vi "ncAFM Amplitude Calibration.vi"() -> ()   [LabVIEW 2021]
doc: "This example calculates the amplitude calibration in non-contact AFM mode.\n\nThis routine is explained in detail in the \"Automated Amplitude Calibration In non-contact AFM\" application note which can be found in www.specs-zurich.com.\n\n\n- Nanonis Programming Interface -"
uses:
  Nanonis Prog Interface.lvlib
  <vilib>/Analysis/NI_AALPro.lvlib
  <vilib>/Analysis/NI_AALBase.lvlib
  <vilib>/Utility/config.llb/NI_LVConfig.lvlib
  <vilib>/Utility/config.llb/Write Key (Double).vi
  Instance           1 35Saved   ncAFM Amplitude Calibration .vi
panel:
  out "Initial P-gain":sgl
  in  "Finish":bool
  in  "apply calib":bool
  out "Initial Z-Controller\nsetpoint [Hz]":sgl format="%.2p"
  out "Initial amplitude A [m]":sgl format="%.2p"
  in  "Tip lift [m]":sgl format="%.2p"
  out "Standard deviation":dbl format="%.2p"
  out "Mean calibration  [m/V]":dbl format="%.2p"
  out "Calibration":cluster{i32[], dbl[]}(graph)
  in  "No. sweeps":i32
  in  "DA [m]":dbl format="%.2p"
  out "Initial calibration [m/V]":sgl format="%.2p"
  in  "Choose PLL":enum16{"PLL1", "PLL2"}(ring)=enum."PLL2"
  in  "No. Points":i32=10
  out "Z versus Amplitude":cluster{dbl[], "Best Linear Fit":dbl[]}[](graph)
  out "Gamma":dbl format="%.2p"
  in  "Machine name (localhost)":string="localhost"
  # "Amplitude calibration in nc-AFM\n\nUser input parameters:  The user should set up the PLL before the calibration procedure.  The amplitude setpoint in Oscillator Controller (A) and the setpoint of the Z-controller (Df) have to be setup to  values the user used to work with (approach or scan). Then the desired PLL has to be selected (useful for Dual-OC4 users).  The maximum amplitude range for sweeping the amplitude has to be also specified by the users (A±DA). \"no. Points\" defines the sweeping points for the amplitude in the range 2DA, and \"no of sweeps\" is the repetition number of the sweeping process.  When the calibration is calculated and applied the tip has to be lifted up; the user has to set in the begining the \"Tip lift\".\nMake sure the tip is engaged and then run the vi.\n\nRead initial settings: The program returns the actual amplitude (A) , the current calibration,  the current Df and calculates the changing factor gamma.\n\nAveraged calibration:  After the calibration procedure is repeated \" no. sweeps\" times , the mean calibration [m/V]  and the standard deviation are returned.\nWhen the mean calibration is calculated the user has to press either the \"Apply calibration\" button or the \"Finish\" button.\n\nThis routine is explained in detail in the \"Automated Amplitude Calibration In non-contact AFM\" application note which can be found in the Applications section of www.specs-zurich.com."
  # "User input parameters"
  # "Read initial settings"
  # "Averaged calibration"
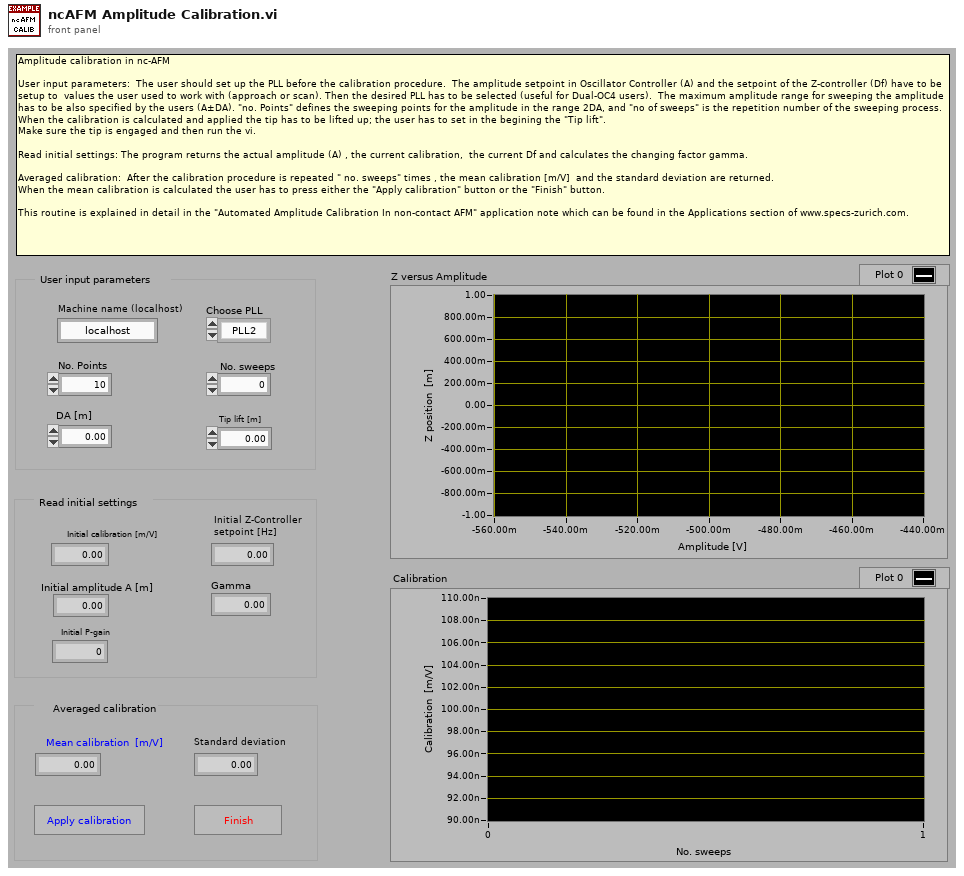
[diagram p1: front panel]
types:
  T1 = typedef "NI_LVConfig.lvlib/Config Data RefNum.ctl" = refnum<k1>
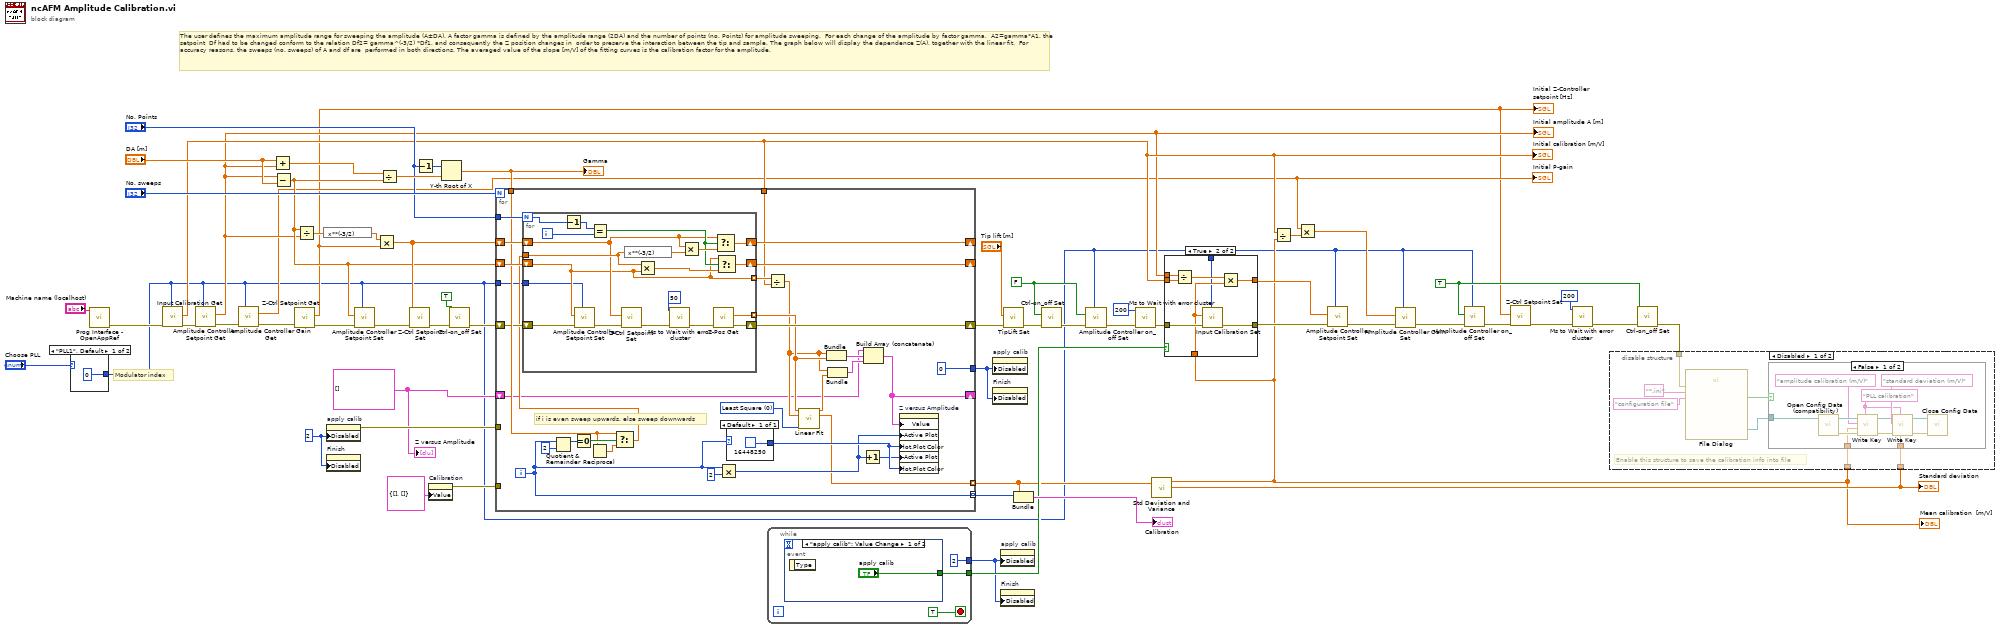
[diagram p0: block diagram]
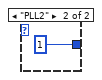
[diagram p2: hidden frame]
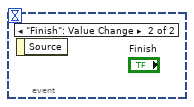
[diagram p5: hidden frame]
diagram:
  w40 = u8 2 ("Disabled")
  w27 = cluster{dbl[], "Best Linear Fit":dbl[]}[] [] ("appended array")
  w18 = TRUE
  w19 = FALSE
  # "Modulator index"
  # "The user defines the maximum amplitude range for sweeping the amplitude (A±DA). A factor gamma is defined by the amplitude range (2DA) and the number of points (no. Points) for amplitude sweeping.  For each change of the amplitude by factor gamma,  A2=gamma*A1, the setpoint  Df had to be changed conform to the relation Df2= gamma^(-3/2) *Df1, and consequently the Z position changes in  order to preserve the interaction between the tip and sample. The graph below will display the dependence Z(A), together with the linear fit.  For accuracy reasons, the sweeps (no. sweeps) of A and df are  performed in both directions. The averaged value of the slope [m/V] of the fitting curves is the calibration factor for the amplitude."
  n1 = case shown="\"PLL1\", Default" "Choose PLL" {
    tunnel: [0 ("Modulator index") 1 ("Modulator index")] -> w3
    frame "PLL1", Default {
    }
    frame "PLL2" {
    }
  }
  n2 = call <userlib>:"Prog Interface - OpenAppRef.vi"("Machine name (local machine IP)"="Machine name (localhost)") -> ("Error out"=w16:errorcluster)  [unwired: 5 in, 1 out]
  n3 = call <userlib>:"Input Calibration Get.vi"("Modulator index"=w3, "Error in (no error)"=w16) -> ("Error out"=w4:errorcluster, "Calibration (m/V)"=w15:sgl)  [unwired: 7 in, 1 out]
  "Initial calibration [m/V]" <- w15
  n4 = call <userlib>:"Amplitude Controller Setpoint Get.vi"("Modulator index"=w3, "Error in (no error)"=w4) -> ("Error out"=w5:errorcluster, "Amplitude (m)"=w14:sgl)  [unwired: 7 in, 1 out]
  "Initial amplitude A [m]" <- w14
  n5 = call <userlib>:"Amplitude Controller Gain Get.vi"("Modulator index"=w3, "Error in (no error)"=w5) -> ("P-gain (V/m)"=w13:sgl, "Error out"=w17:errorcluster)  [unwired: 9 in, 3 out]
  "Initial P-gain" <- w13
  n6 = Add(x="DA [m]", y=w14) -> (x+y=w48:dbl)
  n7 = Subtract(x=w14, y="DA [m]") -> (x-y=w34:dbl)
  n8 = call <userlib>:"Z-Ctrl Setpoint Get.vi"("error in (no error)"=w17) -> ("error out"=w44:errorcluster, "Z Controller setpoint"=w10:sgl)  [unwired: 7 in, 1 out]
  "Initial Z-Controller\nsetpoint [Hz]" <- w10
  n9 = Divide(x=w34, y=w14) -> (x/y=w47:dbl)
  n10 = expression code="x**(-3/2)"(w47) -> (w46:dbl)
  n11 = property on="apply calib" class="Bool"("Disabled"=w40) -> (error out=w39:errorcluster)  [unwired: 2 in, 1 out]
  n12 = property on="Finish" class="Bool"("Disabled"=w40) -> ()  [unwired: 2 in, 2 out]
  n13 = call <userlib>:"Amplitude Controller Setpoint Set.vi"("Modulator index"=w3, "Error in (no error)"=w44, "Amplitude (m)"=w34) -> ("Error out"=w45:errorcluster)  [unwired: 7 in, 1 out]
  n14 = Multiply(x=w46, y=w10) -> (x*y=w43:dbl)
  n15 = Divide(x=w48, y=w34) -> (x/y=w57:dbl)
  n16 = call <userlib>:"Z-Ctrl Setpoint Set.vi"("error in (no error)"=w45, "Z Controller setpoint"=w43) -> ("error out"=w60:errorcluster)  [unwired: 8 in, 1 out]
  n17 = Decrement(x="No. Points") -> (x-1=w56:i32)
  n18 = property on="Calibration" class="XYGraph (strict)"("Value"=cluster{i32[], dbl[]} {[], []} ("Calibration")) -> (error out=w25:errorcluster)  [unwired: 2 in, 1 out]
  n19 = Y-th Root of X(1:w57, 2:w56) -> (0:w55:dbl)
  "Gamma" <- w55
  n20 = call <userlib>:"Ctrl-on_off Set.vi"("error in (no error)"=w60, "Z Controller ON/OFF"=TRUE) -> ("error out"=w31:errorcluster)  [unwired: 8 in, 1 out]
  n21 = for {
    N: "No. sweeps" -> [_]
    tunnel: "No. Points" -> [w89]
    tunnel: w55 -> [w84]
    shift-right: [w81] -> w29
    shift-left: w31 -> [w80]
    shift-right: [w78] -> _
    shift-left: w43 -> [w90]
    shift-right: [w77] -> _
    shift-left: w34 -> [w88]
    tunnel: w15 -> [w75]
    shift-right: [w67] -> _
    shift-left: w27 -> [w72]
    tunnel: w39 -> [_]
    tunnel: [u8 0 ("Disabled")] -> w38
    tunnel: [w65] -> w36 mode=indexing
    tunnel: [w64] -> w35 mode=indexing
    tunnel: w25 -> [_]
    tunnel: w3 -> [w63]
    i -> [w65]
    w91 = u16 0 items=["Least Square", "Least Absolute Residual", "Bisquare"] ("method")
    # "if i is even sweep upwards, else sweep downwards"
    n22 = Quotient & Remainder(x=w65, y=2) -> (x-y*floor(x/y)=w86:i32)  [unwired: 1 out]
    n23 = Equal To 0?(x=w86) -> (x = 0?=w85:bool)
    n24 = Reciprocal(x=w84) -> (1/x=w83:dbl)
    n25 = Select(t=w84, s=w85, f=w83) -> (s? t:f=w79:dbl)
    n26 = for {
      N: w89 -> [w109]
      tunnel: w79 -> [w112]
      shift-right: [w114] -> w81
      shift-left: w80 -> [w111]
      shift-right: [w102] -> w77
      shift-left: w88 -> [w99]
      shift-right: [w105] -> w78
      shift-left: w90 -> [w101]
      tunnel: [w100] -> w74 mode=indexing
      tunnel: [w99] -> w76 mode=indexing
      tunnel: w63 -> [w95]
      i -> [w108]
      n27 = Decrement(x=w109) -> (x-1=w107:i32)
      n28 = call <userlib>:"Amplitude Controller Setpoint Set.vi"("Modulator index"=w95, "Error in (no error)"=w111, "Amplitude (m)"=w99) -> ("Error out"=w110:errorcluster)  [unwired: 7 in, 1 out]
      n29 = Equal?(x=w107, y=w108) -> (x = y?=w104:bool)
      n30 = call <userlib>:"Z-Ctrl Setpoint Set.vi"("error in (no error)"=w110, "Z Controller setpoint"=w101) -> ("error out"=w97:errorcluster)  [unwired: 8 in, 1 out]
      n31 = expression code="x**(-3/2)"(w112) -> (w113:dbl)
      n32 = Multiply(x=w112, y=w99) -> (x*y=w103:dbl)
      n33 = call "Ms to Wait with error cluster.vi"("error in (no error)"=w97, "milliseconds to wait"=u32 50) -> ("error out"=w96:errorcluster)  [unwired: 4 in, 1 out]
      n34 = Multiply(x=w101, y=w113) -> (x*y=w106:dbl)
      n35 = call <userlib>:"Z-Pos Get.vi"("error in (no error)"=w96) -> ("error out"=w114:errorcluster, "Z position (m)"=w100:sgl)  [unwired: 8 in, 1 out]
      n36 = Select(t=w101, s=w104, f=w106) -> (s? t:f=w105:dbl)
      n37 = Select(t=w99, s=w104, f=w103) -> (s? t:f=w102:dbl)
    }
    n38 = Multiply(x=w65, y=2) -> (x*y=w69:i32)
    n39 = case shown="Default" w65 {
      tunnel: [u32 16448250] -> w71
      frame Default {
      }
    }
    n40 = Divide(x=w76, y=w75) -> (x/y=w73:dbl[])
    n41 = call <vilib>:"Linear Fit.vi"("Y"=w74, "X"=w73, "method"=w91) -> ("Best Linear Fit"=w82:dbl[], "slope"=w64:dbl)  [unwired: 8 in, 3 out]
    n42 = Bundle(w73, w74) -> (w92:cluster{dbl[], sgl[]})  [unwired: 1 in]
    n43 = Bundle(w73, "Best Linear Fit"=w82) -> (w93:cluster{dbl[], "Best Linear Fit":dbl[]})  [unwired: 1 in]
    n44 = Increment(x=w69) -> (x+1=w68:i32)
    n45 = Build Array (concatenate)(w72, w92, w93) -> (w67:cluster{dbl[], "Best Linear Fit":dbl[]}[])
    n46 = property on="Z versus Amplitude" class="XYGraph (strict)"("Value"=w67, "Active Plot"=w69, "Plot.Plot Color"=w71, "Active Plot"=w68, "Plot.Plot Color"=w71) -> ()  [unwired: 2 in, 2 out]
  }
  n47 = while {
    tunnel: [w116] -> w41
    tunnel: [u8 2 ("Disabled")] -> w37
    stop <- TRUE stop-if-true
    n48 = event shown="[0] \"apply calib\": Value Change" {
      selector: _ -> [_ _]
      dyn-events: _ -> [_ _]
      timeout: _ -> [_ _]
      tunnel: ["apply calib" _] -> w116
      event "apply calib": Value Change {
        n49 = event-data() -> ()  [unwired: 1 in, 1 out]
      }
      event "Finish": Value Change {
        n50 = event-data() -> ()  [unwired: 1 in, 1 out]
      }
    }
  }
  n51 = property on="apply calib" class="Bool"("Disabled"=w38) -> ()  [unwired: 2 in, 2 out]
  n52 = property on="Finish" class="Bool"("Disabled"=w38) -> ()  [unwired: 2 in, 2 out]
  n53 = property on="apply calib" class="Bool"("Disabled"=w37) -> ()  [unwired: 2 in, 2 out]
  n54 = property on="Finish" class="Bool"("Disabled"=w37) -> ()  [unwired: 2 in, 2 out]
  n55 = call <userlib>:"TipLift Set.vi"("error in (no error)"=w29, "TipLift (m)"="Tip lift [m]") -> ("error out"=w30:errorcluster)  [unwired: 8 in, 1 out]
  n56 = Bundle(w36, w35) -> (→"Calibration":cluster{i32[], dbl[]})  [unwired: 1 in]
  n57 = call <userlib>:"Ctrl-on_off Set.vi"("error in (no error)"=w30, "Z Controller ON/OFF"=w19) -> ("error out"=w21:errorcluster)  [unwired: 8 in, 1 out]
  n58 = call <userlib>:"Amplitude Controller on_off Set.vi"("Modulator index"=w3, "Error in (no error)"=w21, "Amplitude controller ON/OFF"=w19) -> ("Error out"=w20:errorcluster)  [unwired: 7 in, 1 out]
  n59 = call "Ms to Wait with error cluster.vi"("error in (no error)"=w20, "milliseconds to wait"=u32 200) -> ("error out"=w51:errorcluster)  [unwired: 4 in, 1 out]
  n60 = call <vilib>:"Std Deviation and Variance.vi"("X"=w35) -> ("mean"=w24:dbl, "standard deviation"=w53:dbl)  [unwired: 1 in, 1 out]
  "Mean calibration  [m/V]" <- w24
  "Standard deviation" <- w53
  n61 = case shown="True" w41 {
    tunnel: w51 -> [w120 w128]
    tunnel: [w120 w127] -> w52
    tunnel: w24 -> [_ w125]
    tunnel: [w119 w124] -> w42
    tunnel: w14 -> [w119 w123]
    tunnel: w15 -> [_ w122]
    tunnel: w3 -> [_ w121]
    frame False {
    }
    frame True {
      n62 = Divide(x=w123, y=w122) -> (x/y=w126:sgl)
      n63 = call <userlib>:"Input Calibration Set.vi"("Modulator index"=w121, "Error in (no error)"=w128, "Calibration (m/V)"=w125) -> ("Error out"=w127:errorcluster)  [unwired: 7 in, 1 out]
      n64 = Multiply(x=w126, y=w125) -> (x*y=w124:dbl)
    }
  }
  n65 = Divide(x=w15, y=w24) -> (x/y=w23:dbl)
  n66 = Multiply(x=w13, y=w23) -> (x*y=w22:dbl)
  n67 = call <userlib>:"Amplitude Controller Setpoint Set.vi"("Modulator index"=w3, "Error in (no error)"=w52, "Amplitude (m)"=w42) -> ("Error out"=w2:errorcluster)  [unwired: 7 in, 1 out]
  n68 = call <userlib>:"Amplitude Controller Gain Set.vi"("Modulator index"=w3, "Error in (no error)"=w2, "P-gain (V/m) (NaN=no change)"=w22) -> ("Error out"=w1:errorcluster)  [unwired: 7 in, 1 out]
  n69 = call <userlib>:"Amplitude Controller on_off Set.vi"("Modulator index"=w3, "Error in (no error)"=w1, "Amplitude controller ON/OFF"=w18) -> ("Error out"=w11:errorcluster)  [unwired: 7 in, 1 out]
  n70 = call <userlib>:"Z-Ctrl Setpoint Set.vi"("error in (no error)"=w11, "Z Controller setpoint"=w10) -> ("error out"=w8:errorcluster)  [unwired: 8 in, 1 out]
  n71 = call "Ms to Wait with error cluster.vi"("error in (no error)"=w8, "milliseconds to wait"=u32 200) -> ("error out"=w7:errorcluster)  [unwired: 4 in, 1 out]
  n72 = call <userlib>:"Ctrl-on_off Set.vi"("error in (no error)"=w7, "Z Controller ON/OFF"=w18) -> ("error out"=w12:errorcluster)  [unwired: 8 in, 1 out]
  n73 = disable-structure shown="Disabled" {
    disable-tunnel: w53 -> [w135 _]
    disable-tunnel: w24 -> [w134 _]
    disable-tunnel: w12 -> [w129 _]
    frame Disabled {
      # "Enable this structure to save the calibration info into file"
      n74 = call "File Dialog"("error in"=w129, "pattern (all files)"="*.ini", "pattern label"="configuration file") -> ("selected path"=w133:path, "cancelled"=w132:bool)  [unwired: 9 in, 2 out]
      n75 = case shown="False" w132 {
        tunnel: w133 -> [w147 _]
        tunnel: w135 -> [w137 _]
        tunnel: w134 -> [w136 _]
        frame False {
          w141 = "PLL calibration" ("section")
          n76 = call <vilib>:"Open Config Data (compatibility).vi"("configuration file path"=w147) -> ("error out"=w146:errorcluster, "refnum"=w145:T1)  [unwired: 8 in, 1 out]
          n77 = call-poly <vilib>:"Write Key.vi"("section"=w141, "error in (no error)"=w146, "value"=w136, "key"="amplitude calibration (m/V)", "refnum"=w145) -> ("error out"=w143:errorcluster, "refnum out"=w138:T1)  [unwired: 4 in, 1 out]
          n78 = call-poly <vilib>:"Write Key.vi"("section"=w141, "error in (no error)"=w143, "value"=w137, "key"="standard deviation (m/V)", "refnum"=w138) -> ("error out"=w140:errorcluster, "refnum out"=w139:T1)  [unwired: 4 in, 1 out]
          n79 = call <vilib>:"Close Config Data.vi"("error in (no error)"=w140, "refnum"=w139) -> ()  [unwired: 8 in, 2 out]
        }
        frame True {
        }
      }
    }
    frame Enabled {
    }
  }
  "Z versus Amplitude" <- w27
